vi "DisplayProperties.vi"(11 "Class In":refnum<class "NiPxi6123.lvclass">) -> (3 "Class out":refnum<class "NiPxi6123.lvclass">)   [LabVIEW 2014, in "SamplerPlugins.lvlib" / "NiPxi6123.lvclass"]
uses:
  NiPxi6123.lvclass
panel:
  out "TaskDAQmx":string
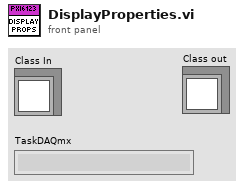
[diagram p1: front panel]
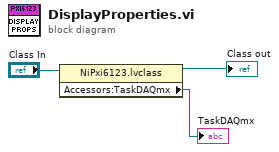
[diagram p0: block diagram]
diagram:
  n1 = property class="NiPxi6123.lvclass"(reference="Class In") -> (reference out=→"Class out":refnum<class "NiPxi6123.lvclass">, "Accessors:TaskDAQmx"=→"TaskDAQmx":refnum<k21>)  [unwired: 1 in, 1 out]
